vi "Default Header.vi"(8 "error in (no error)":errorcluster) -> (0 "error out":errorcluster, 3 "<JSON>":string caption="Default Header <JSON>")   [LabVIEW 2017, in "JSONWebToken.lvclass"]
uses:
  JSONWebToken.lvclass
  header.ctl
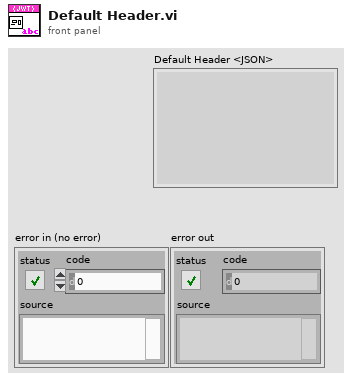
[diagram p1: front panel]
types:
  T1 = typedef "header.ctl" = cluster{"alg":string, "jku":string, "jwk":string, "kid":string, "x5u":string, "x5c":string, "x5t":string, "x5t#S256":string, "typ":string, "cty":string, "crit":string, "enc":string}
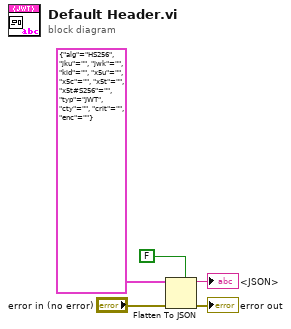
[diagram p0: block diagram]
diagram:
  n1 = Flatten To JSON(enable LabVIEW extensions? (T)=FALSE, anything=T1 {"alg"="HS256", "jku"="", "jwk"="", "kid"="", "x5u"="", "x5c"="", "x5t"="", "x5t#S256"="", "typ"="JWT", "cty"="", "crit"="", "enc"=""} ("header"), error in (no error)="error in (no error)") -> (JSON string=→"<JSON>":string, 11:→"error out":errorcluster)
